vi "GetgitRevision.vi"(11 "File Path Control":path caption="File Path Control (leave blank to use Constants_Global value of EnFlo SW Folder)") -> (0 "This Folder's Last Changed Date":string, 2 "LocalModifications":string, 3 "OverallRevision":string, 4 "standard error":string, 5 "standard output":string)   [LabVIEW 2016]
doc: "This VI uses the system's installed svn (subversion) software to return the revision number of the selected folder. Leaving the selected folder blank will use the global value of \"EnFlo SW Folder\".\nThe \"Overall Revision\" is the highest revision number in the entire hierarchy, recursing upwards as well as downwards- in other words, the revision which was checked out. The \"This Folder\" data is specific to the last changes to the selected folder."
uses:
  Globals/Constants_global.vi
panel:
  out "This Folder Last Committed By":string
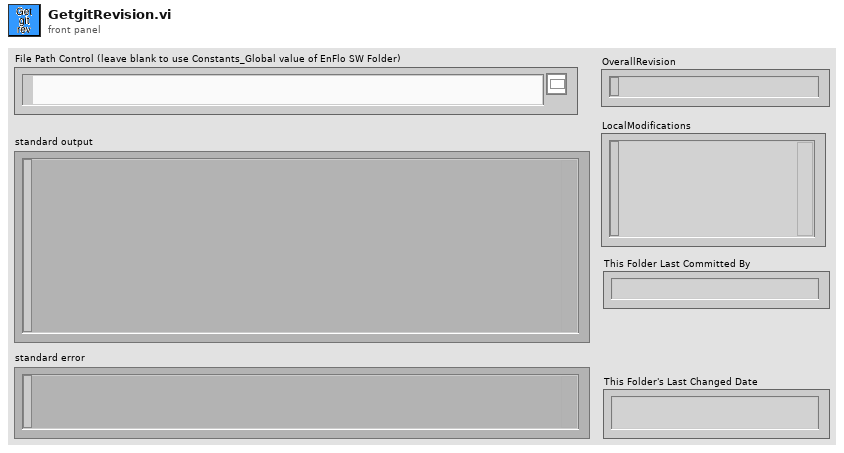
[diagram p1: front panel]
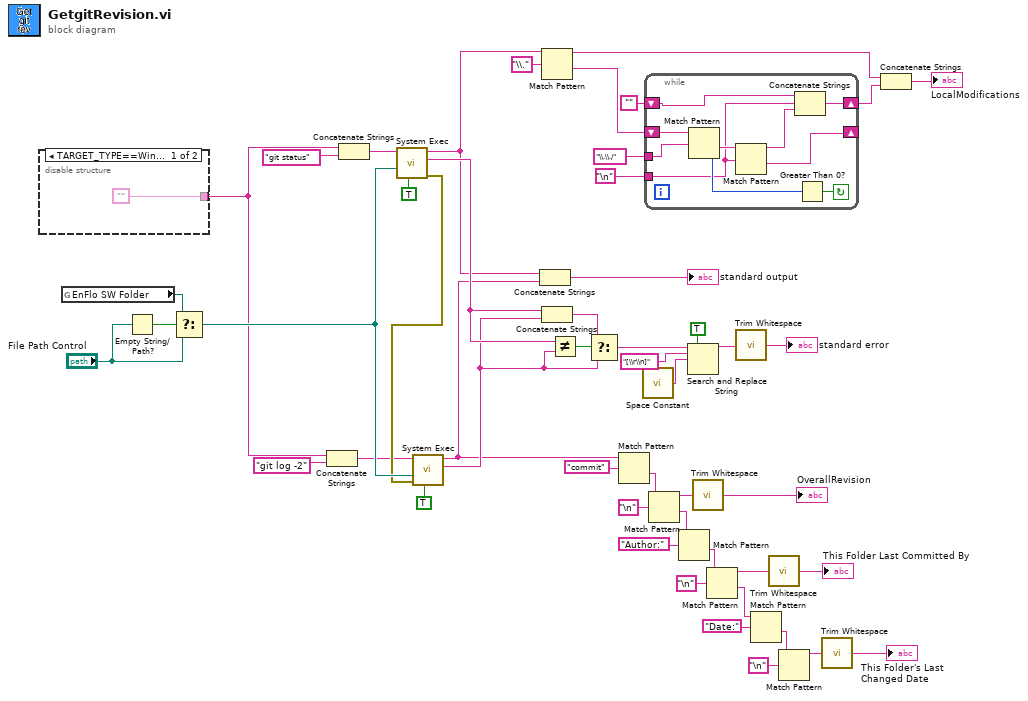
[diagram p0: block diagram]
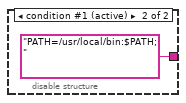
[diagram p2: hidden frame]
diagram:
  n1 = disable-structure shown="TARGET_TYPE==Windows, Default" {
    disable-tunnel: ["" ("command line") "PATH=/usr/local/bin:$PATH; " ("command line")] -> w16
    frame condition #0 {
    }
    frame condition #1 (active) {
    }
  }
  n2 = global read "Constants_global.vi" "EnFlo SW Folder"() -> (w48:path)
  n3 = Empty String/Path?(string/path="File Path Control") -> (empty?=w50:bool)
  n4 = Select(t=w48, s=w50, f="File Path Control") -> (s? t:f=w34:path)
  n5 = Concatenate Strings(w16, "git log -2" ("command line")) -> (w18:string)
  n6 = Concatenate Strings(w16, "git status" ("command line")) -> (w20:string)
  n7 = call <vilib>:"System Exec.vi"("run minimized? (F)"=TRUE, "working directory"=w34, "command line"=w20) -> ("error out"=w32:errorcluster, "standard error"=w29:string, "standard output"=w9:string)  [unwired: 5 in, 1 out]
  n8 = call <vilib>:"System Exec.vi"("run minimized? (F)"=TRUE, "error in (no error)"=w32, "working directory"=w34, "command line"=w18) -> ("standard error"=w26:string, "standard output"=w13:string)  [unwired: 4 in, 2 out]
  n9 = Concatenate Strings(w9, w13) -> (→"standard output":string)
  n10 = Match Pattern(string=w9, regular expression="\\.") -> (before substring=w2:string, after substring=w7:string)  [unwired: 1 in, 2 out]
  n11 = Concatenate Strings(w29, w26) -> (w27:string)
  n12 = Not Equal?(x=w29, y=w26) -> (x != y?=w28:bool)
  n13 = Select(t=w27, s=w28, f=w26) -> (s? t:f=w22:string)
  n14 = Match Pattern(string=w13, regular expression="commit") -> (after substring=w46:string)  [unwired: 1 in, 3 out]
  n15 = call <vilib>:"Space Constant.vi"() -> ("String"=w24:string)
  n16 = while {
    shift-right: [w59] -> _
    shift-left: w7 -> [w62]
    tunnel: "\\.\\./" -> [w61]
    tunnel: "\n" -> [w54]
    shift-right: [w55] -> w3
    shift-left: "" -> [w53]
    stop <- w57 continue-if-true
    n17 = Match Pattern(string=w62, regular expression=w61) -> (after substring=w60:string, offset past match=w58:i32)  [unwired: 1 in, 2 out]
    n18 = Match Pattern(string=w60, regular expression=w54) -> (before substring=w56:string, after substring=w59:string)  [unwired: 1 in, 2 out]
    n19 = Concatenate Strings(w53, w54, w56) -> (w55:string)
    n20 = Greater Than 0?(x=w58) -> (x > 0?=w57:bool)
  }
  n21 = Match Pattern(string=w46, regular expression="\n") -> (before substring=w44:string, after substring=w43:string)  [unwired: 1 in, 2 out]
  n22 = Match Pattern(string=w43, regular expression="Author:") -> (after substring=w40:string)  [unwired: 1 in, 3 out]
  n23 = Search and Replace String(replace all?=TRUE ("replace all? (F)"), input string=w22, search string="[\\r\\n]", replace string=w24) -> (result string=w21:string)  [unwired: 4 in, 3 out]
  n24 = call <vilib>:"Trim Whitespace.vi"("string"=w44) -> ("trimmed string"=→"OverallRevision":string)  [unwired: 1 in]
  n25 = Match Pattern(string=w40, regular expression="\n") -> (before substring=w39:string, after substring=w12:string)  [unwired: 1 in, 2 out]
  n26 = call <vilib>:"Trim Whitespace.vi"("string"=w21) -> ("trimmed string"=→"standard error":string)  [unwired: 1 in]
  n27 = Match Pattern(string=w12, regular expression="Date:") -> (after substring=w37:string)  [unwired: 1 in, 3 out]
  n28 = call <vilib>:"Trim Whitespace.vi"("string"=w39) -> ("trimmed string"=→"This Folder Last Committed By":string)  [unwired: 1 in]
  n29 = Match Pattern(string=w37, regular expression="\n") -> (before substring=w35:string)  [unwired: 1 in, 3 out]
  n30 = call <vilib>:"Trim Whitespace.vi"("string"=w35) -> ("trimmed string"=→"This Folder's Last Changed Date":string)  [unwired: 1 in]
  n31 = Concatenate Strings(w2, w3) -> (→"LocalModifications":string)
